vi "Read.vi"(8 "error in (no error)":errorcluster, 11 "Subset_STR in":refnum<class "Insert_STR.lvclass">) -> (0 "error out":errorcluster, 2 "String":string, 3 "Subset_STR out":refnum<class "Insert_STR.lvclass">)   [LabVIEW 2021, in "Insert_STR.lvclass"]
uses:
  Insert_STR.lvclass
  Insert_STR.lvclass/Insert_STR.ctl
  Abs_Types/String/Abs_String.lvclass
  Abs_Types/Numeric/Abs_Numeric.lvclass
  Abs_Types/Value/Abs_Value.lvclass
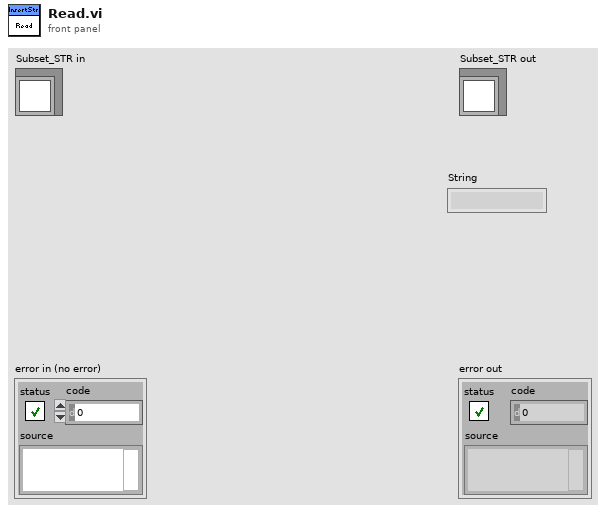
[diagram p1: front panel]
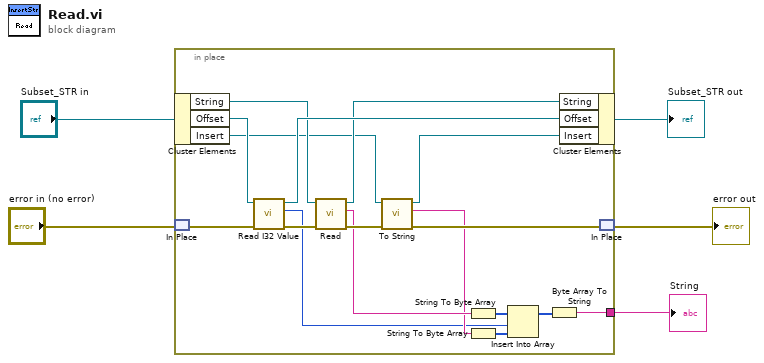
[diagram p0: block diagram]
diagram:
  n1 = in-place {
    in-place-border: [w9] -> w3
    n2 = in-place-cluster #1("Subset_STR in") -> ("String"=w18:refnum<class "Abs_String.lvclass">, "Offset"=w20:refnum<class "Abs_Numeric.lvclass">, "Insert"=w15:refnum<class "Abs_Value.lvclass">)
    n3 = in-place-match #2("error in (no error)") -> (w22:errorcluster)
    n4 = call-dynamic "Read I32 Value.vi"("error in (no error)"=w22, "Numeric in"=w20) -> ("error out"=w21:errorcluster, "I32"=w6:i32, "Numeric out"=w19:refnum<class "Abs_Numeric.lvclass">)  [unwired: 7 in]
    n5 = call-dynamic "Read.vi"("error in (no error)"=w21, "Abs_String in"=w18) -> ("error out"=w16:errorcluster, "String"=w8:string, "Abs_String out"=w17:refnum<class "Abs_String.lvclass">)  [unwired: 7 in]
    n6 = call-dynamic "To String.vi"("error in (no error)"=w16, "Types in"=w15) -> ("error out"=w13:errorcluster, "String"=w7:string, "Types out"=w14:refnum<class "Abs_Value.lvclass">)  [unwired: 7 in]
    n7 = String To Byte Array(string=w8) -> (unsigned byte array=w10:u8[])
    n8 = String To Byte Array(string=w7) -> (unsigned byte array=w11:u8[])
    n9 = Insert Into Array(array=w10, index=w6, new element=w11) -> (w12:u8[])
    n10 = Byte Array To String(unsigned byte array=w12) -> (string=w9:string)
    n11 = in-place-cluster #1("String"=w17, "Offset"=w19, "Insert"=w14) -> (→"Subset_STR out":refnum<class "Insert_STR.lvclass">)
    n12 = in-place-match #2(w13) -> (→"error out":errorcluster)
  }
  "String" <- w3
